vi "ROIlistautofill.vi"(7 "ROI in (pix)":i32=60 min=0 step=2, 8 "error out":errorcluster, 9 "ImageName":string=".jpg", 10 "bead array in":u32[][](array[numeric]), 11 "ImagePath":string="data path") -> (0 "error out 2":errorcluster, 1 "Bead Array":i32[][](array[numeric]), 2 "Reg of Int of the bead":u8[][](graph), 3 "ROI center list":i32[][](array[numeric]), 4 "ROI out":i32=40)   [LabVIEW 2011, in "OfflineTracker.lvlib"]
uses:
  OfflineTracker.lvlib
  <vilib>/Utility/file.llb/Write To Spreadsheet File (I64).vi
panel:
  in  "ROI (pix)":i32=80
  in  "Proximity\n (ROI size units)":dbl=0.4
  out "Beads Found":i32
  in  "Acceptance range":dbl=0.25 step=0.01
  in  "Autofind?":bool=TRUE
  in  "stop":bool
  out "ori image":u8[][](graph)
  in  "Reset all":bool
  in  "Remove":bool
  in  "Add bead":bool
  # "page up"
  # "page down"
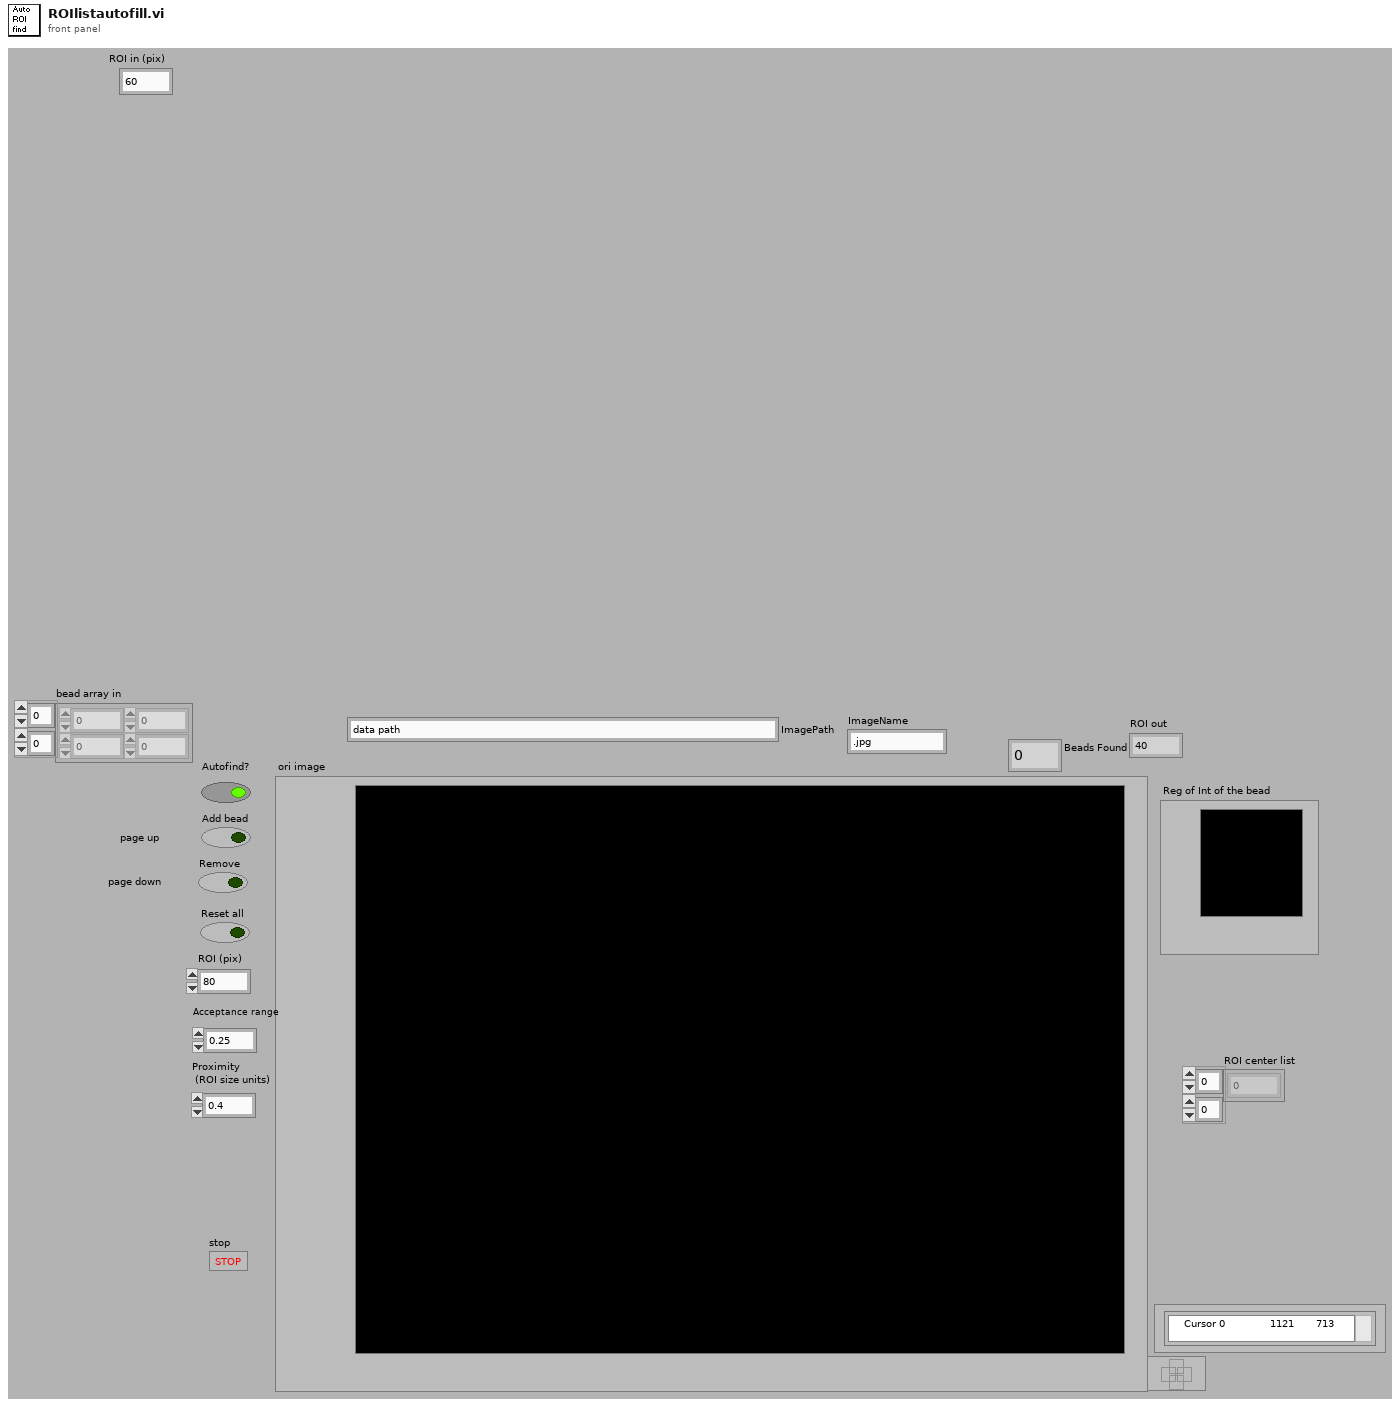
[diagram p1: front panel]
types:
  T1 = typedef "IMAQ Image.ctl" = refnum<image>
  T2 = typedef "LVPointDoubleTypeDef.ctl" = cluster{"Cursor X":dbl, "Cursor Y":dbl}
  T3 = cluster{"front panel settings":cluster{"files":cluster{"LUT path":path, "Trace path":path, " folders #":i32, "base path":path, "use trace":bool, "use base":bool, "LUT tmp":i32, "Trace tmp":i32, "active path":path}, "Tracking":cluster{"RminZ (pix)":i32, "Rmax (pix)":i32, "angular pixel \ncoverage factor":dbl, "radial pixel \ncoverage factor":dbl}, "Frames":cluster{"Start frame":i32, "number of frames":u32, "display frame ":i32, "track every nd frame ":i32, "Track all frames":bool, "active frame":i32}, "Calibs":cluster{"Zlut number of steps":i32, "pix/um":dbl, "Z correction factor":dbl, "Zlut step size (um)":dbl, "ROI(pix)":i32}, "Beads":cluster{"number of ref beads":i32, "overlay":bool}, "Misc":cluster{"save images to new location":bool, "destination":path}}, "data":cluster{"Image":T1, "image size":i32[], "Bead Array":i32[][], "overlay image":T1, "# beads":i32, "Job list":string[][], "job running":bool, "job #":i32, "folders to go":i32}}
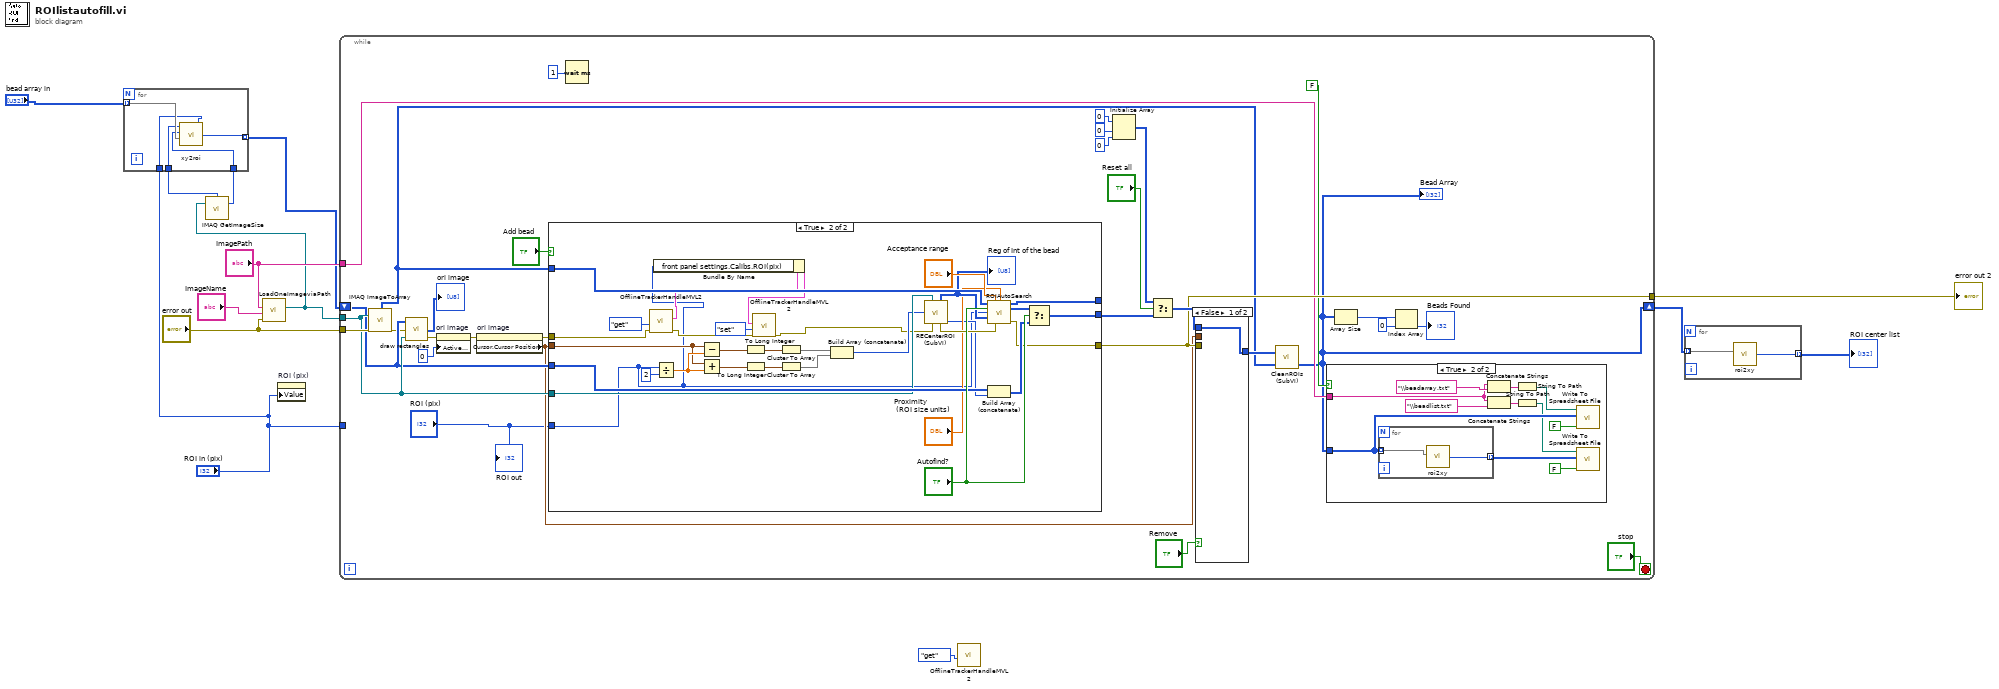
[diagram p0: block diagram]
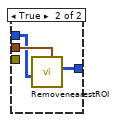
[diagram p3: hidden frame]
diagram:
  n1 = call "LoadOneImageviaPath.vi"("ImagePath"="ImagePath", "ImageName"="ImageName", "error in (no error)"="error out") -> ("Image Out"=w4:T1)  [unwired: 7 out]
  n2 = call "IMAQ GetImageSize"("Image"=w4) -> ("Y Resolution"=w2:i32, "X Resolution"=w3:i32)  [unwired: 3 in, 1 out]
  n3 = for {
    tunnel: "bead array in" -> [w18] mode=indexing
    tunnel: [w17] -> w5 mode=indexing
    tunnel: "ROI in (pix)" -> [w16]
    tunnel: w3 -> [w15]
    tunnel: w2 -> [w14]
    n4 = call "xy2roi.vi"("ROI1"=w16, "xy"=w18, "Y Resolution"=w14, "X Resolution"=w15) -> ("ROI"=w17:i32[])  [unwired: 1 in, 1 out]
  }
  n5 = property on="ROI (pix)" class="DigNum (strict)"("Value"="ROI in (pix)") -> ()  [unwired: 2 in, 2 out]
  n6 = while {
    tunnel: "error out" -> [w39]
    tunnel: [w38] -> w8
    shift-right: [w20] -> w11
    shift-left: w5 -> [w36]
    tunnel: w4 -> [w37]
    tunnel: "ImagePath" -> [w22]
    tunnel: "ROI in (pix)" -> [_]
    stop <- "stop" stop-if-true
    n7 = call "IMAQ ImageToArray"("error in (no error)"=w39, "Image"=w37) -> ("error out"=w35:errorcluster, "Image Pixels (U8)"=w21:u8[][])  [unwired: 1 in, 4 out]
    n8 = call "draw rectangles.vi"("Image"=w37, "error in (no error)"=w35, "Array"=w36) -> ("error out"=w26:errorcluster, "Image Pixels (U8)"=→"ori image":u8[][])  [unwired: 1 out]
    n9 = property on="ori image" class="IntGraph (strict)"(error in=w26, "Active Cursor"=u32 0) -> (error out=w29:errorcluster)  [unwired: 1 in, 1 out]
    n10 = property on="ori image" class="IntGraph (strict)"(error in=w29) -> (error out=w27:errorcluster, "Cursor.Cursor Position"=w25:T2)  [unwired: 1 in, 1 out]
    n11 = case shown="True" "Add bead" {
      tunnel: w37 -> [_ w84]
      tunnel: [w68 w90] -> w41
      tunnel: w36 -> [w68 w86]
      tunnel: [w67 w83] -> w38
      tunnel: w21 -> [_ w88]
      tunnel: [w68 w85] -> _
      tunnel: w25 -> [_ w79]
      tunnel: w27 -> [w67 w75]
      tunnel: "ROI (pix)" -> [_ w69]
      frame False {
      }
      frame True {
        n12 = call "OfflineTrackerHandleMVL2.vi"("error in"=w75, "action"=enum16{"get", "set"}."get") -> ("error out"=w74:errorcluster, "out"=w72:T3)  [unwired: 4 in]
        n13 = Bundle By Name(cluster=w72, "front panel settings.Calibs.ROI(pix)"=w69) -> (w71:T3)
        n14 = Divide(x=w69, y=2) -> (x/y=w97:dbl)
        n15 = Subtract(x=w79, y=w97) -> (x-y=w99:T2)
        n16 = Add(x=w79, y=w97) -> (x+y=w98:T2)
        n17 = To Long Integer(number=w99) -> (32bit integer=w96:cluster{"Cursor X":i32, "Cursor Y":i32})
        n18 = To Long Integer(number=w98) -> (32bit integer=w94:cluster{"Cursor X":i32, "Cursor Y":i32})
        n19 = call "OfflineTrackerHandleMVL2.vi"("error in"=w74, "action"=enum16{"get", "set"}."set", "in"=w71) -> ("error out"=w73:errorcluster)  [unwired: 3 in, 1 out]
        n20 = Cluster To Array(cluster=w96) -> (array=w95:i32[])
        n21 = Cluster To Array(cluster=w94) -> (array=w93:i32[])
        n22 = Build Array (concatenate)(w95, w93) -> (w78:i32[])
        n23 = call "RECenterROI (SubVI).vi"("Image in"=w84, "ROI in LTRB"=w78, "error out 2"=w73) -> ("Imageout"=w82:u8[][], "LTRB improved"=w77:u32[], "error out"=w81:errorcluster)  [unwired: 10 out]
        "Reg of Int of the bead" <- w82
        n24 = call "ROIAutoSearch.vi"("multi image in"=w88, "Correlation \nTreshold\n(0..1)"="Acceptance range", "Proximity (ROI size units)"="Proximity\n (ROI size units)", "Autofind?"="Autofind?", "ROI (pix)"=w69, "template image in"=w82, "error out"=w81) -> ("Reg of Int of the bead 2"=w85:u8[][], "ROI array out"=w87:u32[][], "error out 3"=w83:errorcluster)  [unwired: 1 in, 5 out]
        n25 = Build Array (concatenate)(w86, w77) -> (w91:u32[][])
        n26 = Select(t=w87, s="Autofind?", f=w91) -> (s? t:f=w90:u32[][])
      }
    }
    n27 = Wait (ms)(milliseconds to wait=u32 1) -> ()  [unwired: 1 out]
    n28 = Initialize Array(0 ("element"), 0 ("dimension size"), 0 ("dimension size")) -> (w44:i32[][])
    n29 = Select(t=w44, s="Reset all", f=w41) -> (s? t:f=w42:u32[][])
    n30 = case shown="False" "Remove" {
      tunnel: [w63 w65] -> w24
      tunnel: w42 -> [w63 w64]
      tunnel: w38 -> [_ _]
      tunnel: w25 -> [_ w66]
      frame False {
      }
      frame True {
        n31 = call "RemovenearestROI.vi"("Cursor.Cursor Position"=w66, "ROI array in"=w64) -> ("ROI array out 2"=w65:u32[][])  [unwired: 8 out]
      }
    }
    n32 = call "CleanROIs (SubVI).vi"("Image Pixels (U8) 2"=w21, "ROI array out 3"=w24) -> ("ROI array out 2"=w20:u32[][])  [unwired: 1 out]
    "Bead Array" <- w20
    n33 = case shown="True" FALSE ("Saving ROIlist") {
      tunnel: w20 -> [_ w56]
      tunnel: w22 -> [_ w51]
      frame False {
      }
      frame True {
        n34 = for {
          tunnel: w56 -> [w62] mode=indexing
          tunnel: [w61] -> w50 mode=indexing
          n35 = call "roi2xy.vi"("ROI"=w62) -> ("xy"=w61:i32[])  [unwired: 5 out]
        }
        n36 = Concatenate Strings(w51, "\\beadarray.txt") -> (w58:string)
        n37 = Concatenate Strings(w51, "\\beadlist.txt") -> (w53:string)
        n38 = String To Path(string=w58) -> (path=w57:path)
        n39 = String To Path(string=w53) -> (path=w52:path)
        n40 = call-poly <vilib>:"Write To Spreadsheet File.vi"("append to file? (new file:F)"=FALSE, "2D data"=w56, "file path (dialog if empty)"=w57) -> ()  [unwired: 3 in, 3 out]
        n41 = call-poly <vilib>:"Write To Spreadsheet File.vi"("append to file? (new file:F)"=FALSE, "2D data"=w50, "file path (dialog if empty)"=w52) -> ()  [unwired: 3 in, 3 out]
      }
    }
    n42 = Array Size(array=w20) -> (size(s)=w34:i32[])
    n43 = Index Array(array=w34, index=0) -> (element=→"Beads Found":i32)
    "ROI out" <- "ROI (pix)"
  }
  "error out 2" <- w8
  n44 = call "OfflineTrackerHandleMVL2.vi"("action"=enum16{"get", "set"}."get") -> ()  [unwired: 5 in, 2 out]
  n45 = for {
    tunnel: w11 -> [w102] mode=indexing
    tunnel: [w101] -> w10 mode=indexing
    n46 = call "roi2xy.vi"("ROI"=w102) -> ("xy"=w101:i32[])  [unwired: 5 out]
  }
  "ROI center list" <- w10
